vi "checkTimeout.vi"(8 "error in (no error)":errorcluster, 10 "ElectrometerController in":refnum<class "ElectrometerController.lvclass">, 11 "UntilIntensityReading in":refnum<class "UntilIntensityReading.lvclass">) -> (0 "error out":errorcluster, 1 "timeout?":bool, 2 "ElectrometerController out":refnum<class "ElectrometerController.lvclass">, 3 "UntilIntensityReading out":refnum<class "UntilIntensityReading.lvclass">)   [LabVIEW 2016, in "UntilIntensityReading.lvclass"]
uses:
  UntilIntensityReading.lvclass
  ElectrometerController/ElectrometerController.lvclass
  Electrometer.lvclass
  ElectrometerConfiguration/ElectrometerInternalConfiguration.lvclass
  State.lvclass
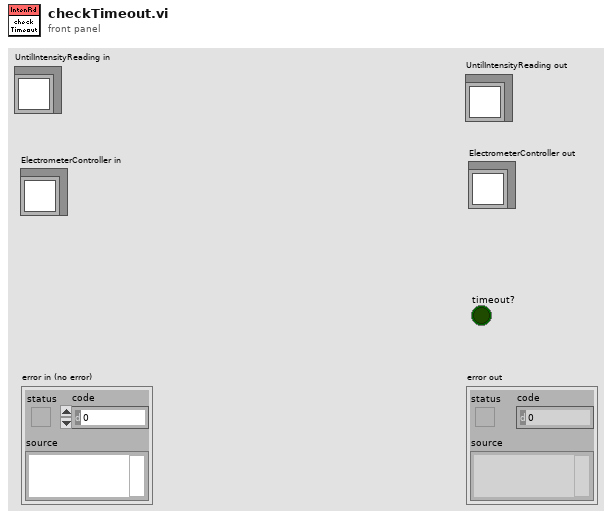
[diagram p1: front panel]
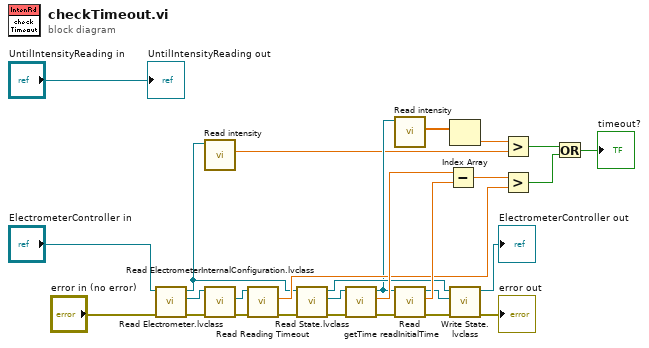
[diagram p0: block diagram]
diagram:
  n1 = call-dynamic "Read Electrometer.lvclass.vi"("error in (no error)"="error in (no error)", "ElectrometerController in"="ElectrometerController in") -> ("error out"=w25:errorcluster, "Electrometer.lvclass"=w28:refnum<class "Electrometer.lvclass">, "ElectrometerController out"=w7:refnum<class "ElectrometerController.lvclass">)  [unwired: 7 in]
  n2 = call-dynamic "Read intensity.vi"("ElectrometerController in"=w7) -> ("intensity"=w2:dbl)  [unwired: 8 in, 2 out]
  n3 = call-dynamic "Read ElectrometerInternalConfiguration.lvclass.vi"("error in (no error)"=w25, "Electrometer in"=w28) -> ("error out"=w26:errorcluster, "ElectrometerInternalConfiguration.lvclass"=w27:refnum<class "ElectrometerInternalConfiguration.lvclass">)  [unwired: 7 in, 1 out]
  n4 = call-dynamic "Read Reading Timeout.vi"("error in (no error)"=w26, "ElectrometerInternalConfiguration in"=w27) -> ("error out"=w21:errorcluster, "Reading Timeout"=w14:dbl)  [unwired: 7 in, 1 out]
  n5 = call-dynamic "Read State.lvclass.vi"("error in (no error)"=w21, "ElectrometerController in"=w7) -> ("error out"=w19:errorcluster, "State.lvclass"=w20:refnum<class "State.lvclass">, "ElectrometerController out"=w16:refnum<class "ElectrometerController.lvclass">)  [unwired: 7 in]
  n6 = call-dynamic "getTime.vi"("error in (no error)"=w19, "State in"=w20) -> ("error out"=w24:errorcluster, "relative seconds"=w23:dbl, "State out"=w4:refnum<class "State.lvclass">)  [unwired: 7 in]
  n7 = call-dynamic "Read intensity.vi"("State in"=w4) -> ("intensity"=w3:dbl[])  [unwired: 8 in, 2 out]
  n8 = call-dynamic "Read readInitialTime.vi"("error in (no error)"=w24, "State in"=w4) -> ("error out"=w18:errorcluster, "readInitialTime"=w22:dbl, "State out"=w17:refnum<class "State.lvclass">)  [unwired: 7 in]
  n9 = Subtract(x=w23, y=w22) -> (x-y=w15:dbl)
  n10 = Index Array(array=w3) -> (element=w1:dbl)  [unwired: 1 in]
  n11 = call-dynamic "Write State.lvclass.vi"("error in (no error)"=w18, "State.lvclass"=w17, "ElectrometerController in"=w16) -> ("error out"=→"error out":errorcluster, "ElectrometerController out"=→"ElectrometerController out":refnum<class "ElectrometerController.lvclass">)  [unwired: 7 in]
  n12 = Greater?(x=w1, y=w2) -> (0:w5:bool)
  n13 = Greater?(x=w15, y=w14) -> (0:w6:bool)
  n14 = Or(x=w5, y=w6) -> (x .or. y?=→"timeout?":bool)
  "UntilIntensityReading out" <- "UntilIntensityReading in"
